vi "_PC_Pub getSequenceFileList.vi"(5 "extention name? (T)":bool=TRUE, 7 "pattern":string="*.*", 8 "error in (no error)":errorcluster, 11 "folderPath":path) -> (0 "error out":errorcluster, 3 "listDataName":string[](array[string]))   [LabVIEW 2018]
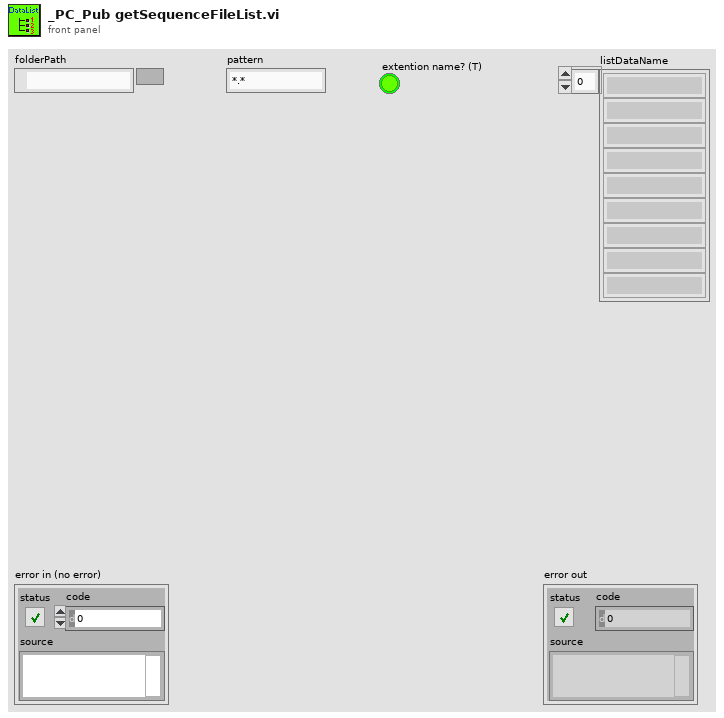
[diagram p1: front panel]
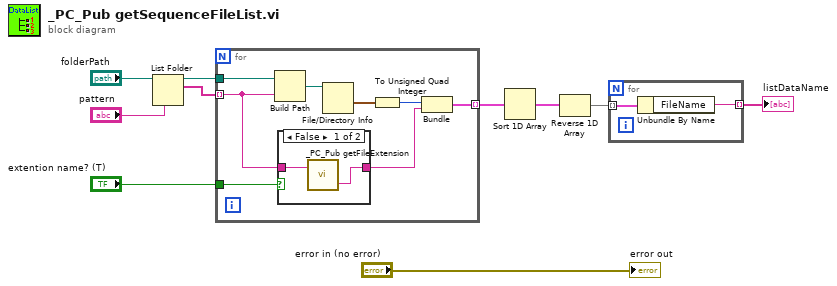
[diagram p0: block diagram]
diagram:
  n1 = List Folder(path="folderPath", pattern="pattern") -> (path out=w5:path, filenames=w8:string[])  [unwired: 2 in, 2 out]
  n2 = for {
    tunnel: w8 -> [w16] mode=indexing
    tunnel: "extention name? (T)" -> [w18]
    tunnel: w5 -> [w17]
    tunnel: [w13] -> w4 mode=indexing
    n3 = Build Path(base path=w17, name or relative path=w16) -> (appended path=w15:path)
    n4 = case shown="False" w18 {
      tunnel: w16 -> [w20 w21]
      tunnel: [w19 w21] -> w12
      frame False {
        n5 = call "_PC_Pub getFileExtension.vi"("Input"=w20) -> ("FileName"=w19:string)  [unwired: 1 in, 1 out]
      }
      frame True {
      }
    }
    n6 = File/Directory Info(path=w15) -> (last mod=w11:timestamp)  [unwired: 1 in, 6 out]
    n7 = To Unsigned Quad Integer(1:w11) -> (0:w14:u64)
    n8 = Bundle(w14, "FileName"=w12) -> (w13:cluster{u64, "FileName":string})  [unwired: 1 in]
  }
  n9 = Sort 1D Array(array=w4) -> (sorted array=w3:cluster{u64, "FileName":string}[])
  n10 = Reverse 1D Array(array=w3) -> (reversed array=w2:cluster{u64, "FileName":string}[])
  n11 = for {
    tunnel: w2 -> [w23] mode=indexing
    tunnel: [w22] -> w1 mode=indexing
    n12 = Unbundle By Name(w23) -> ("FileName"=w22:string)
  }
  "listDataName" <- w1
  "error out" <- "error in (no error)"
